vi "Export Test Case.vi"(8 "error in (no error)":errorcluster, 10 "Test Case":T1, 11 "Node in":refnum<k20>) -> (0 "error out":errorcluster, 3 "Node out":refnum<k20>)   [LabVIEW 2013, in "JUnit for Azure Pipelines.lvclass"]
uses:
  JUnit for Azure Pipelines.lvclass
  Test Case.ctl
  Test Result.ctl
  <vilib>/xml/Close Reference(Node).vi
  <vilib>/xml/NI_XML.lvlib
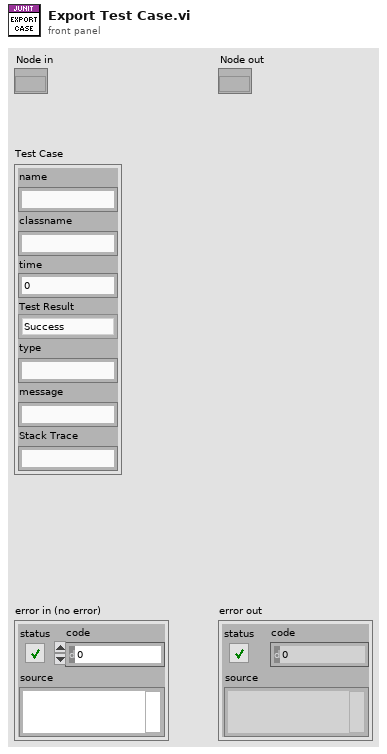
[diagram p1: front panel]
types:
  T1 = typedef "JUnit for Azure Pipelines.lvclass/Test Case.ctl" = cluster{"name":string, "classname":string, "time":dbl, "Test Result":T2, "type":string, "message":string, "Stack Trace":string}
  T2 = typedef "JUnit for Azure Pipelines.lvclass/Test Result.ctl" = enum16{"Success", "Failure", "Error", "Skipped"}
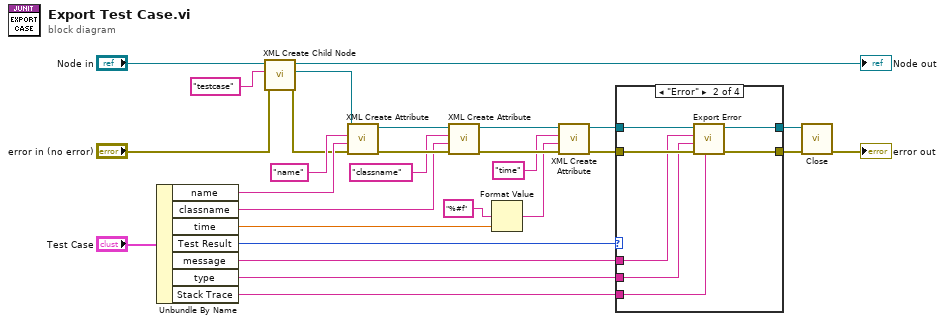
[diagram p0: block diagram]
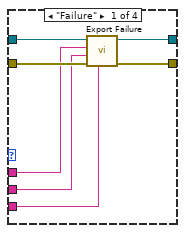
[diagram p2: hidden frame]
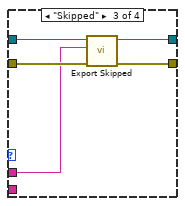
[diagram p3: hidden frame]
diagram:
  n1 = Unbundle By Name("Test Case") -> ("name"=w21:string, "classname"=w11:string, "time"=w10:dbl, "Test Result"=w8:T2, "message"=w5:string, "type"=w4:string, "Stack Trace"=w1:string)
  n2 = call "XML Create Child Node.vi"("error in (no error)"="error in (no error)", "Element Name"="testcase" ("Tag Name"), "Node in"="Node in") -> ("error out"=w12:errorcluster, "Child Node"=w13:refnum<k20>, "Node out"=→"Node out":refnum<k20>)  [unwired: 6 in]
  n3 = call "XML Create Attribute.vi"("error in (no error)"=w12, "Attribute Value"=w21, "Attribute Name"="name", "Node in"=w13) -> ("error out"=w19:errorcluster, "Node out"=w20:refnum<k20>)  [unwired: 6 in]
  n4 = call "XML Create Attribute.vi"("error in (no error)"=w19, "Attribute Value"=w11, "Attribute Name"="classname", "Node in"=w20) -> ("error out"=w16:errorcluster, "Node out"=w17:refnum<k20>)  [unwired: 6 in]
  n5 = Format Value(format string="%#f", value (0)=w10) -> (output string=w9:string)  [unwired: 1 in]
  n6 = call "XML Create Attribute.vi"("error in (no error)"=w16, "Attribute Value"=w9, "Attribute Name"="time", "Node in"=w17) -> ("error out"=w2:errorcluster, "Node out"=w3:refnum<k20>)  [unwired: 6 in]
  n7 = case shown="\"Error\"" w8 {
    tunnel: w3 -> [w35 w42 w47 w49]
    tunnel: [w34 w41 w46 w49] -> w7
    tunnel: [w33 w40 w45 w48] -> w6
    tunnel: w2 -> [w32 w39 w44 w48]
    tunnel: w5 -> [w31 w38 w43 _]
    tunnel: w4 -> [w30 w37 _ _]
    tunnel: w1 -> [w29 w36 _ _]
    frame "Failure" {
      n8 = call "Export Failure.vi"("Stack Trace"=w29, "error in (no error)"=w32, "Type"=w30, "Message"=w31, "Node in"=w35) -> ("error out"=w33:errorcluster, "Node out"=w34:refnum<k20>)  [unwired: 5 in]
    }
    frame "Error" {
      n9 = call "Export Error.vi"("Stack Trace"=w36, "error in (no error)"=w39, "Type"=w37, "Message"=w38, "Node in"=w42) -> ("error out"=w40:errorcluster, "Node out"=w41:refnum<k20>)  [unwired: 5 in]
    }
    frame "Skipped" {
      n10 = call "Export Skipped.vi"("error in (no error)"=w44, "Message"=w43, "Node in"=w47) -> ("error out"=w45:errorcluster, "Node out"=w46:refnum<k20>)  [unwired: 7 in]
    }
    frame "Success" {
    }
  }
  n11 = call-poly <vilib>:"Close.vi"("error in (no error)"=w6, "node"=w7) -> ("error out"=→"error out":errorcluster)  [unwired: 7 in]
